vi "String to Time Stamp.vi"(1 "input string":string) -> (0 "Time Stamp":timestamp)   [LabVIEW 2023, in "Utilities.lvlib"]
uses:
  Utilities.lvlib
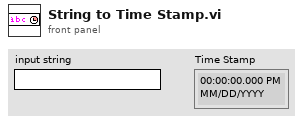
[diagram p1: front panel]
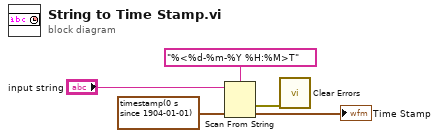
[diagram p0: block diagram]
diagram:
  n1 = Scan From String(format string="%<%d-%m-%Y %H:%M>T", input string="input string", default 1=timestamp(0 s since 1904-01-01)) -> (error out=w1:errorcluster, output 1=→"Time Stamp":timestamp)  [unwired: 2 in, 2 out]
  n2 = call <vilib>:"Clear Errors.vi"("error in (no error)"=w1) -> ()  [unwired: 5 in, 2 out]
